vi "Ethernet Receive.vi"(8 "error in (no error)":errorcluster, 9 "Timeout":i32=5000, 11 "Connection ID":refnum<k5>) -> (0 "error out":errorcluster, 1 "Data":i32 format="%.0x", 2 "Units":string, 3 "Connection ID (dup)":refnum<k5>)   [LabVIEW 2019]
panel:
  # "VI Name: MB Ethernet Receive.vi\nPurpose: Reads a Modbus message over Ethernet.\nReentrant VI, because its caller is also reentrant."
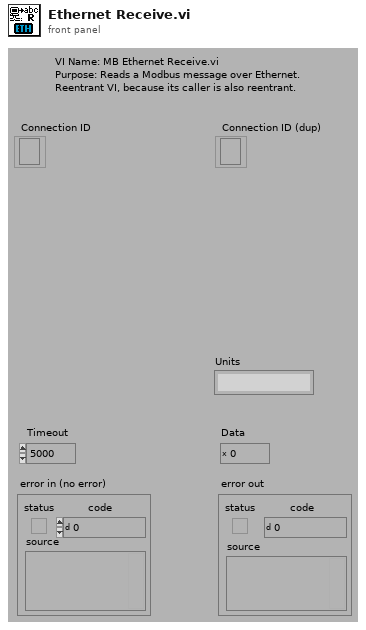
[diagram p1: front panel]
types:
  T1 = enum16{"Standard", "Buffered", "CRLF", "Immediate"}
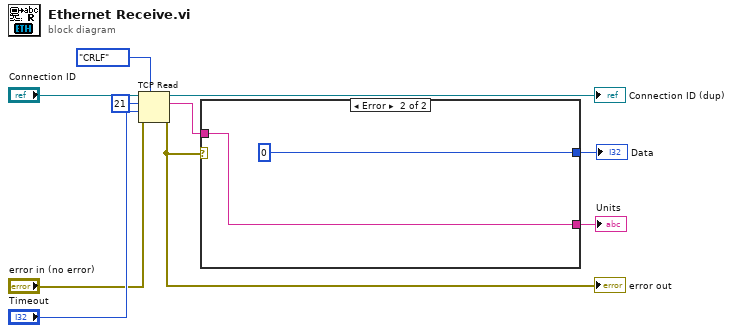
[diagram p0: block diagram]
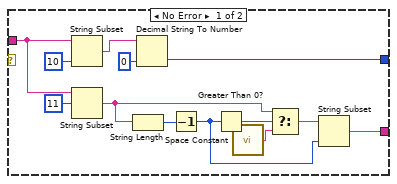
[diagram p2: hidden frame]
diagram:
  n1 = TCP Read(connection ID="Connection ID", bytes to read=21, error in (no error)="error in (no error)", 7:T1."CRLF" ("mode (standard)"), 9:"Timeout") -> (connection ID out=→"Connection ID (dup)":refnum<k5>, data out=w6:string, error out=w4:errorcluster)
  "error out" <- w4
  n2 = case shown="Error" w4 {
    tunnel: w6 -> [w18 w24]
    tunnel: [w22 0] -> w5
    tunnel: [w11 w24] -> w3
    frame No Error {
      n3 = String Subset(string=w18, length (rest)=10 ("length (rest)")) -> (substring=w20:string)  [unwired: 1 in]
      n4 = String Subset(string=w18, offset (0)=11 ("length (rest)")) -> (substring=w16:string)  [unwired: 1 in]
      n5 = String Length(string=w16) -> (length=w14:i32)
      n6 = Decimal String To Number(string=w20, default (0L)=0 ("default (0 I32)")) -> (number=w22:i32)  [unwired: 1 in, 1 out]
      n7 = Decrement(x=w14) -> (x-1=w12:i32)
      n8 = Greater Than 0?(x=w12) -> (x > 0?=w17:bool)
      n9 = call <vilib>:"Space Constant.vi"() -> ("String"=w15:string)
      n10 = Select(t=w16, s=w17, f=w15) -> (s? t:f=w13:string)
      n11 = String Subset(string=w13, length (rest)=w12) -> (substring=w11:string)  [unwired: 1 in]
    }
    frame Error {
    }
  }
  "Data" <- w5
  "Units" <- w3
